vi "Color Rows.vi"(8 "error in (no error)":errorcluster, 11 "DataGrid in":refnum<class "DataGrid.lvclass">) -> (0 "error out":errorcluster, 3 "DataGrid out":refnum<class "DataGrid.lvclass">)   [LabVIEW 2017, in "DataGrid.lvclass"]
uses:
  DataGrid.lvclass
  C:/Program Files (x86)/National Instruments/LabVIEW 2017/vi.lib/QSI/QControls/QControl Classes/Generic/Generic.lvclass
  C:/Program Files (x86)/National Instruments/LabVIEW 2017/vi.lib/QSI/QControls/QControl Classes/MulticolumnListbox/MulticolumnListbox.lvclass
  <vilib>/Utility/miscctls.llb/LVRowAndColumnTypeDef.ctl
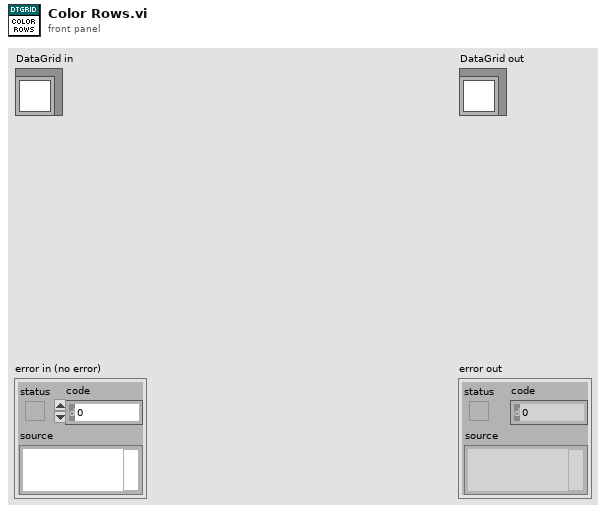
[diagram p1: front panel]
types:
  T1 = typedef "LVRowAndColumnTypeDef.ctl" = cluster{"Row":i32, "Column":i32}
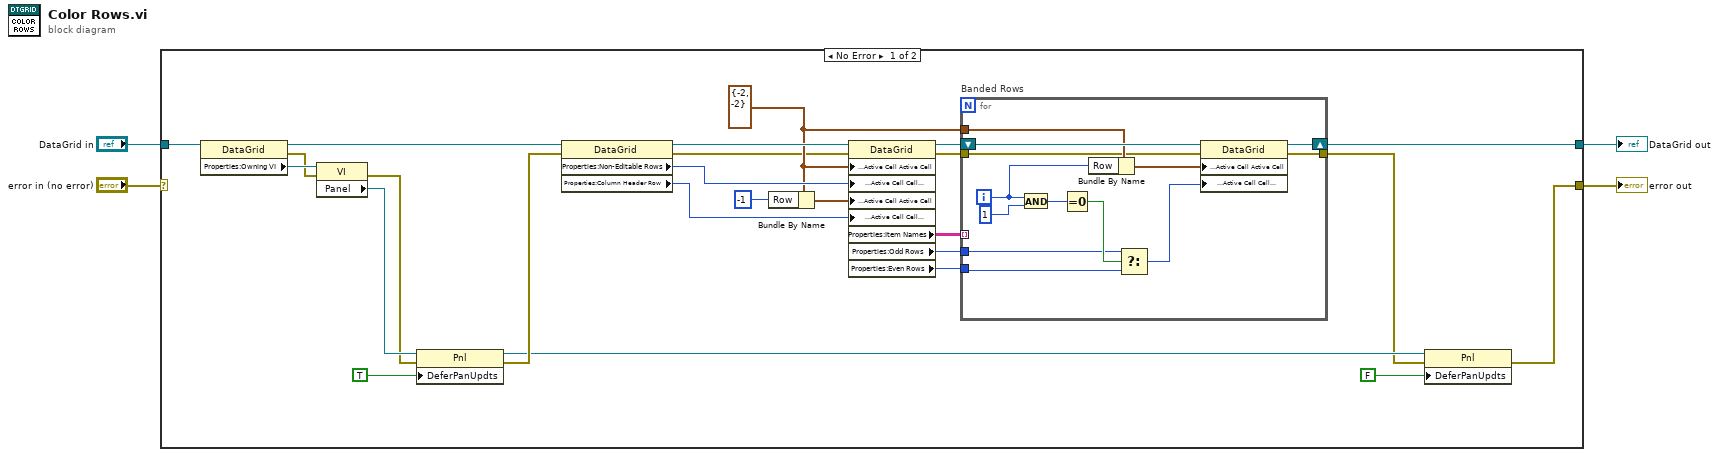
[diagram p0: block diagram]
diagram:
  n1 = case shown="No Error" "error in (no error)" {
    selector: "error in (no error)" -> [_ w44]
    tunnel: [w6 w44] -> w3
    tunnel: [w18 w43] -> w1
    tunnel: "DataGrid in" -> [w29 w43]
    frame No Error {
      w22 = T1 {"Row"=-2, "Column"=-2} ("Active Cell:Active Cell")
      n2 = property class="DataGrid"(reference=w29) -> (reference out=w15:refnum<class "DataGrid.lvclass">, error out=w12:errorcluster, "Properties:Owning VI"=w14:refnum<vi>)  [unwired: 1 in]
      n3 = property class="VI"(reference=w14, error in=w12) -> (error out=w11:errorcluster, "Panel"=w13:refnum<vi>)  [unwired: 1 out]
      n4 = property class="Pnl"(reference=w13, error in=w11, "DeferPanUpdts"=TRUE ("Defer Panel Updates")) -> (reference out=w7:refnum<vi>, error out=w9:errorcluster)
      n5 = property class="DataGrid"(reference=w15, error in=w9) -> (reference out=w28:refnum<class "DataGrid.lvclass">, error out=w17:errorcluster, "Properties:Non-Editable Rows"=w27:u32, "Properties:Column Header Row"=w24:u32)
      n6 = Bundle By Name(cluster=w22, "Row"=-1) -> (w25:T1)
      n7 = property class="DataGrid"(reference=w28, error in=w17, "Properties:Active Cell Active Cell"=w22, "Properties:Active Cell Cell Background Color"=w27, "Properties:Active Cell Active Cell"=w25, "Properties:Active Cell Cell Background Color"=w24) -> (reference out=w23:refnum<class "DataGrid.lvclass">, error out=w16:errorcluster, "Properties:Item Names"=w21:string[][], "Properties:Odd Rows"=w20:u32, "Properties:Even Rows"=w19:u32)
      n8 = for "Banded Rows" {
        tunnel: w22 -> [w41]
        tunnel: w21 -> [_] mode=indexing
        tunnel: w20 -> [w35]
        tunnel: w19 -> [w34]
        shift-right: [w32] -> w18
        shift-left: w23 -> [w42]
        tunnel: w16 -> [w30]
        tunnel: [w31] -> w5
        i -> [w38]
        n9 = And(x=w38, y=1) -> (x .and. y?=w37:i32)
        n10 = Equal To 0?(x=w37) -> (x = 0?=w36:bool)
        n11 = Bundle By Name(cluster=w41, "Row"=w38) -> (w40:T1)
        n12 = Select(t=w35, s=w36, f=w34) -> (s? t:f=w33:u32)
        n13 = property class="DataGrid"(reference=w42, error in=w30, "Properties:Active Cell Active Cell"=w40, "Properties:Active Cell Cell Background Color"=w33) -> (reference out=w32:refnum<class "DataGrid.lvclass">, error out=w31:errorcluster)
      }
      n14 = property class="Pnl"(reference=w7, error in=w5, "DeferPanUpdts"=FALSE ("Defer Panel Updates")) -> (error out=w6:errorcluster)  [unwired: 1 out]
    }
    frame Error {
    }
  }
  "error out" <- w3
  "DataGrid out" <- w1
